vi "Auto cyclic quad ROI.vi"(1 "img_H":i32, 2 "img_W":i32) -> (0 "ROI to crop (pixels)":T1={"Xmax"=2147483647, "Ymax"=2147483647, "Xmin"=0, "Ymin"=0})   [LabVIEW 2015]
uses:
  Typedefs/ROI bounds.ctl
panel:
  # "PN 07/12/2015"
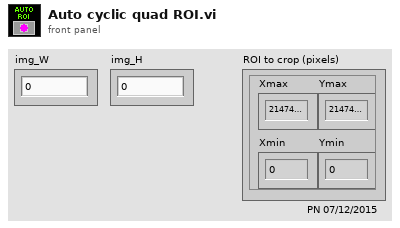
[diagram p1: front panel]
types:
  T1 = typedef "ROI bounds.ctl" = cluster{"Xmax":i32, "Ymax":i32, "Xmin":i32, "Ymin":i32}
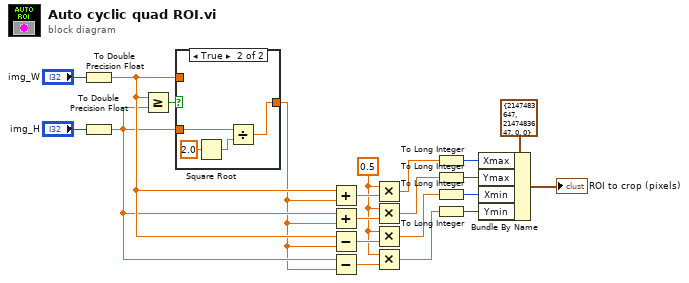
[diagram p0: block diagram]
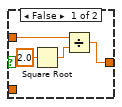
[diagram p2: hidden frame]
diagram:
  w5 = 0.5 ("x")
  n1 = To Double Precision Float(number="img_W") -> (double precision float=w10:dbl)
  n2 = To Double Precision Float(number="img_H") -> (double precision float=w9:dbl)
  n3 = Greater Or Equal?(x=w10, y=w9) -> (x >= y?=w19:bool)
  n4 = case shown="True" w19 {
    tunnel: w10 -> [w23 _]
    tunnel: w9 -> [_ w29]
    tunnel: [w22 w26] -> w8
    frame False {
      n5 = Square Root(x=2.0) -> (sqrt(x)=w25:dbl)
      n6 = Divide(x=w23, y=w25) -> (x/y=w22:dbl)
    }
    frame True {
      n7 = Square Root(x=2.0) -> (sqrt(x)=w28:dbl)
      n8 = Divide(x=w29, y=w28) -> (x/y=w26:dbl)
    }
  }
  n9 = Add(x=w10, y=w8) -> (x+y=w16:dbl)
  n10 = Add(x=w9, y=w8) -> (x+y=w13:dbl)
  n11 = Subtract(x=w10, y=w8) -> (x-y=w7:dbl)
  n12 = Subtract(x=w9, y=w8) -> (x-y=w6:dbl)
  n13 = Multiply(x=w5, y=w16) -> (x*y=w15:dbl)
  n14 = Multiply(x=w5, y=w13) -> (x*y=w12:dbl)
  n15 = Multiply(x=w5, y=w7) -> (x*y=w4:dbl)
  n16 = Multiply(x=w5, y=w6) -> (x*y=w2:dbl)
  n17 = To Long Integer(number=w15) -> (32bit integer=w14:i32)
  n18 = To Long Integer(number=w12) -> (32bit integer=w11:i32)
  n19 = To Long Integer(number=w4) -> (32bit integer=w3:i32)
  n20 = To Long Integer(number=w2) -> (32bit integer=w1:i32)
  n21 = Bundle By Name(cluster=T1 {"Xmax"=2147483647, "Ymax"=2147483647, "Xmin"=0, "Ymin"=0} ("ROI to crop (pixels)"), "Xmax"=w14, "Ymax"=w11, "Xmin"=w3, "Ymin"=w1) -> (→"ROI to crop (pixels)":T1)
